vi "map RGT101 font settings.vi"(1 "font settings  new":T1) -> (0 "font settings  old":T2)   [LabVIEW 2015]
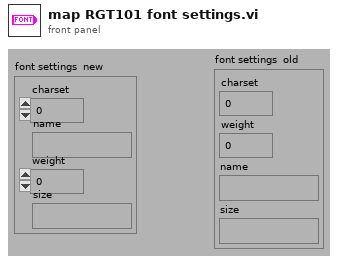
[diagram p1: front panel]
types:
  T1 = cluster{"charset":i16, "name":string, "weight":i16, "size":string}
  T2 = cluster{"charset":i16, "weight":i16, "name":string, "size":string}
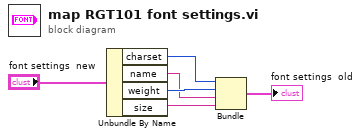
[diagram p0: block diagram]
diagram:
  n1 = Unbundle By Name("font settings  new") -> ("charset"=w4:i16, "name"=w2:string, "weight"=w3:i16, "size"=w1:string)
  n2 = Bundle("charset"=w4, "weight"=w3, "name"=w2, "size"=w1) -> (→"font settings  old":T2)  [unwired: 1 in]
